vi "ReadAndConvertFile.vi"(8 "error in (no error)":errorcluster, 10 "Path":path, 11 "Zero Offset and Degree Transitions in":refnum<class "Zero Offset and Degree Transitions.lvclass">) -> (0 "error out":errorcluster, 2 "EPT Pattern":T1, 3 "Zero Offset and Degree Transitions out":refnum<class "Zero Offset and Degree Transitions.lvclass">)   [LabVIEW 2019, in "File Formats.lvlib" / "Zero Offset and Degree Transitions.lvclass"]
uses:
  Zero Offset and Degree Transitions.lvclass
  Parent/EST Pattern.ctl
  Parent/FileFormat.lvclass
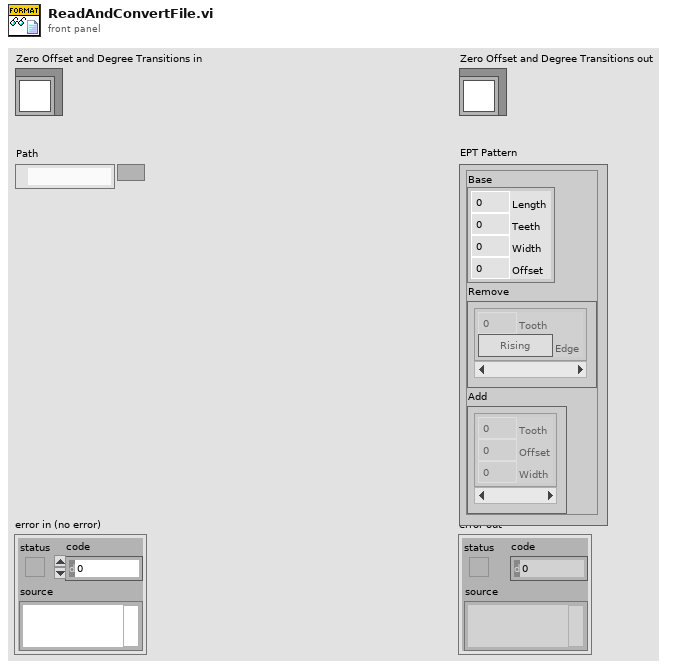
[diagram p1: front panel]
types:
  T1 = typedef "File Formats.lvlib/FileFormat.lvclass/EST Pattern.ctl" = cluster{"Base":cluster{"Length":dbl, "Teeth":u16, "Width":dbl, "Offset":dbl}, "Remove":cluster{"Tooth":u16, "Edge":bool}[], "Add":cluster{"Tooth":u16, "Offset":dbl, "Width":dbl}[]}
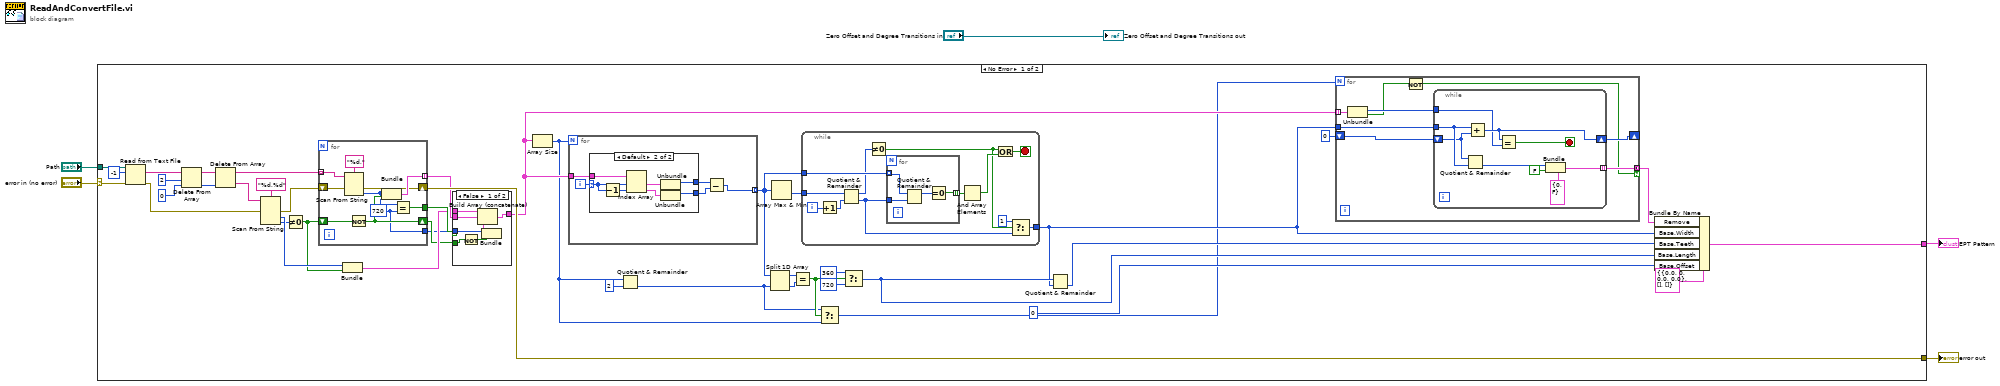
[diagram p0: block diagram]
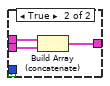
[diagram p2: hidden frame]
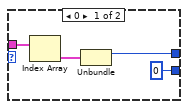
[diagram p3: hidden frame]
diagram:
  n1 = case shown="No Error" "error in (no error)" {
    selector: "error in (no error)" -> [w26 w116]
    tunnel: "Path" -> [w46 _]
    tunnel: [w42 w116] -> w2
    tunnel: [w27 _] -> w1
    frame No Error {
      w41 = 0 ("index")
      n2 = Read from Text File(file (use dialog)=w46, count=-1, error in=w26) -> (text=w43:string[], error out=w36:errorcluster)  [unwired: 1 in, 2 out]
      n3 = Delete From Array(array=w43, length=2, index=w41) -> (array with subset deleted=w40:string[])  [unwired: 1 out]
      n4 = Delete From Array(array=w40, index=w41) -> (deleted portion=w37:string, array with subset deleted=w39:string[])  [unwired: 1 in]
      n5 = Scan From String(format string="%d,%d", input string=w37, error in=w36) -> (error out=w35:errorcluster, output 1=w34:i32, output 2=w30:i32)  [unwired: 3 in, 2 out]
      n6 = Not Equal To 0?(x=w30) -> (x != 0?=w21:bool)
      n7 = for {
        tunnel: w39 -> [w113] mode=indexing
        tunnel: [w115] -> w14 mode=indexing
        shift-right: [w109] -> w12
        shift-left: w21 -> [w110]
        shift-right: [w114] -> w42
        shift-left: w35 -> [w111]
        tunnel: [w107] -> w15
        tunnel: [w106] -> w11
        w106 = 720 ("y")
        n8 = Scan From String(format string="%d,", input string=w113, error in=w111) -> (error out=w114:errorcluster, output 1=w108:i32)  [unwired: 2 in, 2 out]
        n9 = Not(x=w110) -> (.not. x?=w109:bool)
        n10 = Bundle(w108, w109) -> (w115:cluster{i32, bool})  [unwired: 1 in]
        n11 = Equal?(x=w108, y=w106) -> (x = y?=w107:bool)
      }
      n12 = Bundle(w34, w21) -> (w13:cluster{i32, bool})  [unwired: 1 in]
      n13 = case shown="False" w15 {
        tunnel: w14 -> [w52 w56]
        tunnel: w13 -> [w53 w55]
        tunnel: [w51 w54] -> w10
        tunnel: w12 -> [w50 _]
        tunnel: w11 -> [w48 _]
        frame False {
          n14 = Not(x=w50) -> (.not. x?=w49:bool)
          n15 = Bundle("y"=w48, w49) -> (w47:cluster{"y":i32, bool})  [unwired: 1 in]
          n16 = Build Array (concatenate)(w53, w52, w47) -> (w51:cluster{"y":i32, bool}[])
        }
        frame True {
          n17 = Build Array (concatenate)(w55, w56) -> (w54:cluster{i32, bool}[])
        }
      }
      n18 = Array Size(array=w10) -> (size(s)=w7:i32)
      n19 = for {
        N: w7 -> [_]
        tunnel: w10 -> [w94]
        tunnel: [w91] -> w22 mode=indexing
        i -> [w90]
        n20 = case shown="Default" w90 {
          selector: w90 -> [_ w99]
          tunnel: w94 -> [w98 w105]
          tunnel: [w96 w102] -> w93
          tunnel: [0 ("y") w101] -> w92
          frame 0 {
            n21 = Index Array(array=w98) -> (element=w97:cluster{"y":i32, bool})  [unwired: 1 in]
            n22 = Unbundle(w97) -> ("y"=w96:i32)  [unwired: 1 out]
          }
          frame Default {
            n23 = Decrement(x=w99) -> (x-1=w100:i32)
            n24 = Index Array(array=w105, index #1=w99, index #2=w100) -> (element #1=w103:cluster{"y":i32, bool}, element #2=w104:cluster{"y":i32, bool})
            n25 = Unbundle(w103) -> ("y"=w102:i32)  [unwired: 1 out]
            n26 = Unbundle(w104) -> ("y"=w101:i32)  [unwired: 1 out]
          }
        }
        n27 = Subtract(x=w93, y=w92) -> (x-y=w91:i32)
      }
      n28 = Quotient & Remainder(x=w7, y=2) -> (floor(x/y)=w8:i32)  [unwired: 1 out]
      n29 = Split 1D Array(array=w22, index=w8) -> (first subarray=w25:i32[], second subarray=w31:i32[])
      n30 = Array Max & Min(array=w22) -> (min value=w33:i32)  [unwired: 3 out]
      n31 = Equal?(x=w25, y=w31) -> (x = y?=w9:bool)
      n32 = while {
        tunnel: w22 -> [w85]
        tunnel: w33 -> [w82]
        tunnel: [w74] -> w18
        i -> [w81]
        stop <- w78 stop-if-true
        n33 = Increment(x=w81) -> (x+1=w80:i32)
        n34 = Quotient & Remainder(x=w82, y=w80) -> (x-y*floor(x/y)=w79:i32, floor(x/y)=w75:i32)
        n35 = Not Equal To 0?(x=w79) -> (x != 0?=w77:bool)
        n36 = for {
          tunnel: w85 -> [w88] mode=indexing
          tunnel: w75 -> [w89]
          tunnel: [w86] -> w84 mode=indexing
          n37 = Quotient & Remainder(x=w88, y=w89) -> (x-y*floor(x/y)=w87:i32)  [unwired: 1 out]
          n38 = Equal To 0?(x=w87) -> (x = 0?=w86:bool)
        }
        n39 = And Array Elements(Boolean array=w84) -> (logical AND=w83:bool)
        n40 = Compound Arithmetic op=OR(w77, w83) -> (w78:bool)
        n41 = Select(t=1, s=w77, f=w75) -> (s? t:f=w74:i32)
      }
      n42 = Select(t=w8, s=w9, f=w7) -> (s? t:f=w6:i32)
      n43 = Select(t=360, s=w9, f=720) -> (s? t:f=w20:i32)
      n44 = Quotient & Remainder(x=w20, y=w18) -> (floor(x/y)=w24:i32)  [unwired: 1 out]
      n45 = for {
        N: w6 -> [_]
        tunnel: [w62] -> w23 mode=concatenating if=w57
        tunnel: w10 -> [w64] mode=indexing
        shift-right: [w63] -> _
        shift-left: 0 -> [w61]
        tunnel: w18 -> [w60]
        n46 = Unbundle(w64) -> ("y"=w59:i32, w58:bool)
        n47 = Not(x=w58) -> (.not. x?=w57:bool)
        n48 = while {
          tunnel: w59 -> [w67]
          shift-right: [w68] -> w63
          shift-left: w61 -> [w69]
          tunnel: [w72] -> w62 mode=indexing
          tunnel: w60 -> [w70]
          stop <- w66 stop-if-true
          n49 = Quotient & Remainder(x=w69, y=w70) -> (floor(x/y)=w71:i32)  [unwired: 1 out]
          n50 = Add(x=w70, y=w69) -> (x+y=w68:i32)
          n51 = Equal?(x=w68, y=w67) -> (x = y?=w66:bool)
          n52 = Bundle(cluster=cluster{"Tooth":u16, "Edge":bool} {"Tooth"=0, "Edge"=FALSE} ("Cluster"), "Tooth"=w71, "Edge"=FALSE) -> (w72:cluster{"Tooth":u16, "Edge":bool})
        }
      }
      n53 = Bundle By Name(cluster=T1 {"Base"={"Length"=0.0, "Teeth"=0, "Width"=0.0, "Offset"=0.0}, "Remove"=[], "Add"=[]} ("EPT Pattern"), "Remove"=w23, "Base.Width"=w18, "Base.Teeth"=w24, "Base.Length"=w20, "Base.Offset"=0 ("f")) -> (w27:T1)
    }
    frame Error {
    }
  }
  "error out" <- w2
  "EPT Pattern" <- w1
  "Zero Offset and Degree Transitions out" <- "Zero Offset and Degree Transitions in"
